vi "Ramp detection (Max-Min & Mean).vi"(7 "Tolerance":sgl=50.0, 8 "error in (no error)":errorcluster, 10 "Image Dst":T1, 11 "Image Src":T1) -> (0 "error out":errorcluster, 2 "Number of ramp regions":i32, 3 "Image Out":T1)   [LabVIEW 2009]
uses:
  <vilib>/vision/Image Controls.llb/IMAQ Image.ctl
  <vilib>/vision/NI_Vision_Development_Module.lvlib
panel:
  out "Image Out":T1(plugin-control)
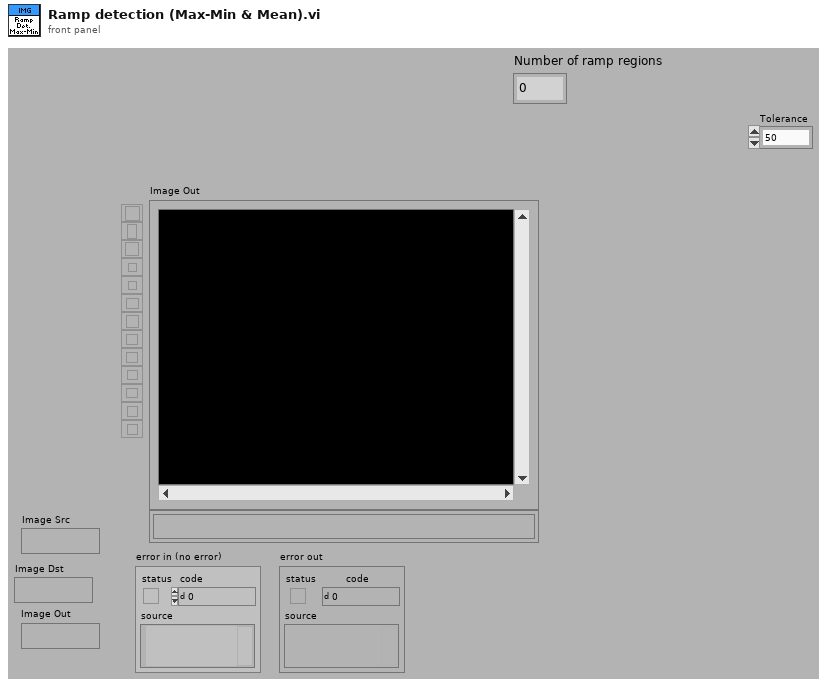
[diagram p1: front panel]
types:
  T1 = typedef "IMAQ Image.ctl" = refnum<image>
  T2 = enum32{"Linear", "Log", "Exp", "Square", "Square root", "Power X", "Power 1/X"}
  T3 = cluster{"Global Rectangle":i32[], "Contours":cluster{"ID":enum32{"External", "Internal"}, "Type":u32, "Coordinates":i32[]}[]}[]
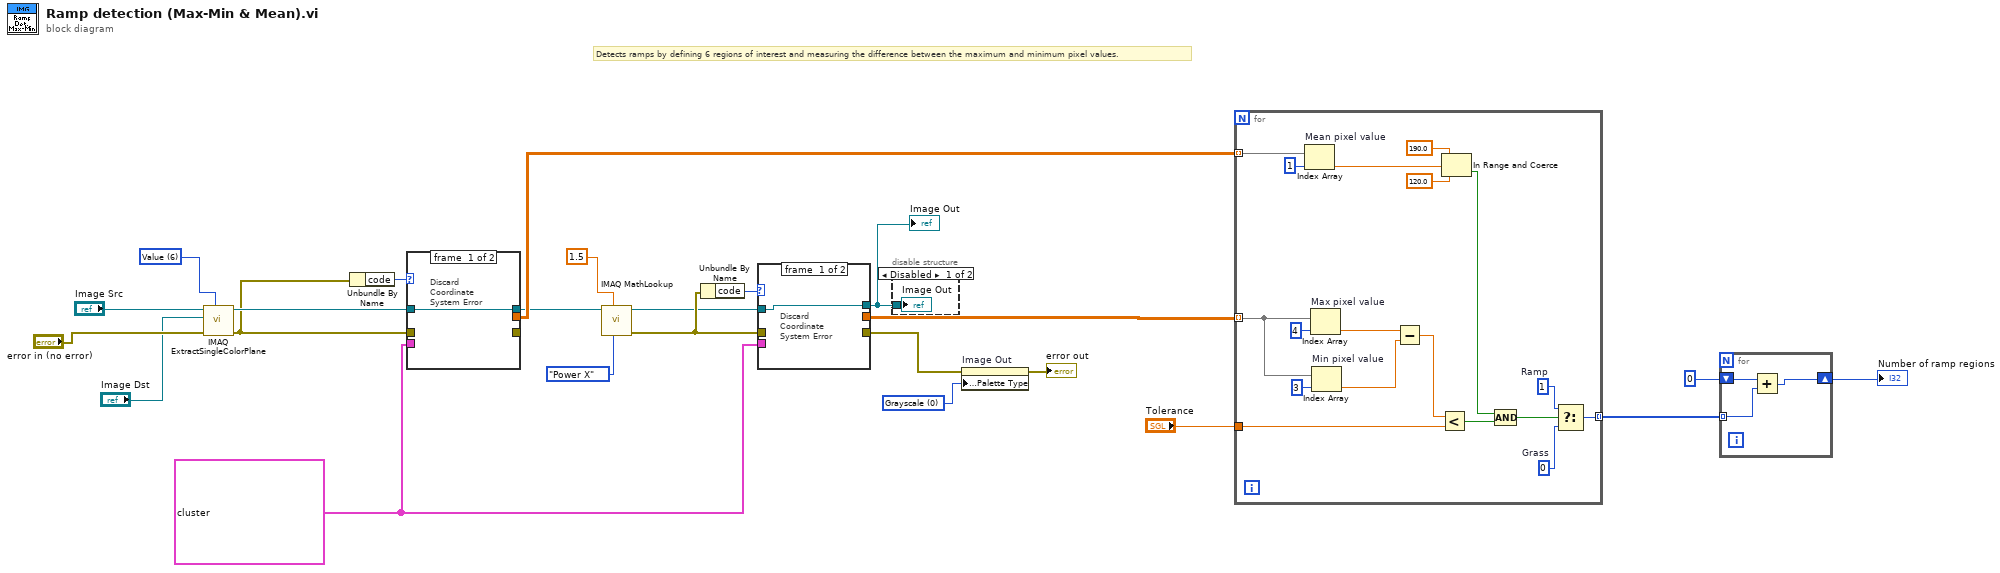
[diagram p0: block diagram]
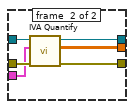
[diagram p2: hidden frame]
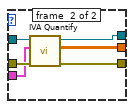
[diagram p4: hidden frame]
diagram:
  w24 = 6 items=["Red", "Green", "Blue", "Hue", "Saturation", "Luminance", "Value", "Intensity"] ("Color Plane (Color Plane Extraction 1)")
  w3 = T3 [{"Global Rectangle"=[18, 13, 28, 23], "Contours"=[{"ID"=enum."External", "Type"=3, "Coordinates"=[18, 13, 28, 23]}]}, {"Global Rectangle"=[77, 13, 87, 23], "Contours"=[{"ID"=enum."External", "Type"=3, "Coordinates"=[77, 13, 87, 23]}]}, {"Global Rectangle"=[135, 12, 145, 23], "Contours"=[{"ID"=enum."External", "Type"=3, "Coordinates"=[135, 12, 145, 23]}]}, {"Global Rectangle"=[18, 53, 28, 64], "Contours"=[{"ID"=enum."External", "Type"=3, "Coordinates"=[18, 53, 28, 64]}]}, {"Global Rectangle"=[77, 53, 87, 64], "Contours"=[{"ID"=enum."External", "Type"=3, "Coordinates"=[77, 53, 87, 64]}]}, {"Global Rectangle"=[137, 54, 146, 64], "Contours"=[{"ID"=enum."External", "Type"=3, "Coordinates"=[137, 54, 146, 64]}]}] ("subarray 2")
  w17 = u32 0 items=["Grayscale", "Binary", "Gradient", "Rainbow", "Temperature", "User Defined"] ("Palette")
  # "Detects ramps by defining 6 regions of interest and measuring the difference between the maximum and minimum pixel values."
  n1 = call "IMAQ ExtractSingleColorPlane"("Color Plane"=w24, "error in (no error)"="error in (no error)", "Image Dst"="Image Dst", "Image Src"="Image Src") -> ("error out"=w4:errorcluster, "Image Dst Out"=w5:T1)  [unwired: 6 out]
  n2 = Unbundle By Name(w4) -> ("code"=w6:i32)
  n3 = case shown="Default" w6 {
    tunnel: [_ w31] -> w2
    tunnel: w5 -> [w25 w30]
    tunnel: w4 -> [_ w29]
    tunnel: [w25 w28] -> w1
    tunnel: [_ w27] -> _
    tunnel: w3 -> [_ w26]
    frame #0 {
      # "Discard\nCoordinate\nSystem Error"
    }
    frame #1 {
      n4 = call <vilib>:"IVA Quantify.vi"("error in (no error)"=w29, "ROI Descriptors"=w26, "Image"=w30) -> ("error out"=w27:errorcluster, "Results"=w31:sgl[][], "Image Out"=w28:T1)  [unwired: 6 out]
    }
  }
  n5 = call "IMAQ MathLookup"("Operator"=T2."Power X" ("Operator (Lookup Table 1)"), "X Value"=sgl 1.5 ("X Value (Lookup Table 1)"), "Image Src"=w1) -> ("error out"=w21:errorcluster, "Image Dst Out"=w20:T1)  [unwired: 4 in, 3 out]
  n6 = Unbundle By Name(w21) -> ("code"=w18:i32)
  n7 = case shown="Default" w18 {
    tunnel: [_ w38] -> w7
    tunnel: w20 -> [w32 w37]
    tunnel: w21 -> [_ w36]
    tunnel: [w32 w35] -> w8
    tunnel: [_ w34] -> w19
    tunnel: w3 -> [_ w33]
    frame #0 {
      # "Discard\nCoordinate\nSystem Error"
    }
    frame #1 {
      n8 = call <vilib>:"IVA Quantify.vi"("error in (no error)"=w36, "ROI Descriptors"=w33, "Image"=w37) -> ("error out"=w34:errorcluster, "Results"=w38:sgl[][], "Image Out"=w35:T1)  [unwired: 6 out]
    }
  }
  "Image Out" <- w8
  n9 = disable-structure shown="Disabled" {
    disable-tunnel: w8 -> [w39 _]
    frame #0 {
      "Image Out" <- w39
    }
    frame #1 {
    }
  }
  n10 = property on="Image Out" class="ImageControl"(error in=w19, "Palette:Palette Type"=w17) -> (error out=→"error out":errorcluster)  [unwired: 1 in, 1 out]
  n11 = for {
    tunnel: w7 -> [w49] mode=indexing
    tunnel: "Tolerance" -> [w53]
    tunnel: [w50] -> w13 mode=indexing
    tunnel: w2 -> [w47] mode=indexing
    w51 = 0  # Grass
    w52 = 1  # Ramp
    n12 = Index Array "Mean pixel value"(array=w47, index=1) -> (element=w45:sgl)
    n13 = Index Array "Max pixel value"(array=w49, index=4) -> (element=w55:sgl)
    n14 = Index Array "Min pixel value"(array=w49, index=3) -> (element=w54:sgl)
    n15 = Subtract(x=w55, y=w54) -> (x-y=w48:sgl)
    n16 = Less?(x=w48, y=w53) -> (x < y?=w41:bool)
    n17 = In Range and Coerce(upper limit=sgl 190.0, x=w45, lower limit=sgl 120.0) -> (In Range?=w40:bool)  [unwired: 1 out]
    n18 = Compound Arithmetic op=AND(w40, w41) -> (w42:bool)
    n19 = Select(t=w52, s=w42, f=w51) -> (s? t:f=w50:i32)
  }
  n20 = for {
    shift-right: [w58] -> w12
    shift-left: 0 ("s? t:f") -> [w60]
    tunnel: w13 -> [w59] mode=indexing
    n21 = Add(x=w60, y=w59) -> (x+y=w58:i32)
  }
  "Number of ramp regions" <- w12
